vi "Lab01_MyFirstVI.2.vi"() -> ()   [LabVIEW 2020]
panel:
  in  "stop":bool
  out "X*X":dbl
  in  "X":dbl
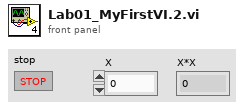
[diagram p1: front panel]
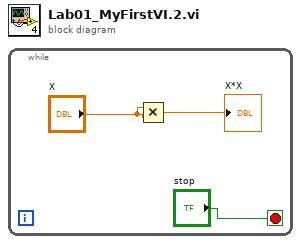
[diagram p0: block diagram]
diagram:
  n1 = while {
    stop <- "stop" stop-if-true
    n2 = Multiply(x="X", y="X") -> (x*y=→"X*X":dbl)
  }
